vi "testRunCalled.vi"() -> (0 "error out":errorcluster)   [LabVIEW 2019, in "TestSuiteTest.lvlib" / "Run.lvlib"]
uses:
  Run/Run.lvlib
  TestSuite/TestSuite.lvclass
  TestCase/TestCase/TestCase.lvclass
  TestSuiteTestSupport/TestResultMock/TestResultMock.lvclass
  C:/Users/de200256/Code/LVUnit/TestResult/TestResult.lvclass
  Assertion/Assertion.lvlib
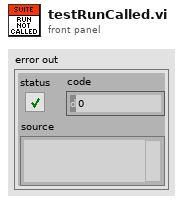
[diagram p1: front panel]
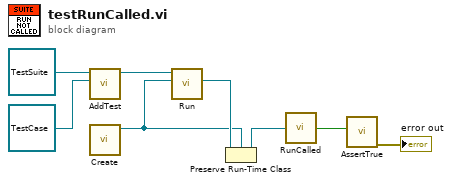
[diagram p0: block diagram]
diagram:
  n1 = call-dynamic "AddTest.vi"("TestCase"=refnum<class "TestCase.lvclass"> refnum, "TestSuite in"=refnum<class "TestSuite.lvclass"> refnum ("TestSuite.lvclass")) -> ("TestSuite out"=w3:refnum<class "TestSuite.lvclass">)  [unwired: 8 in, 1 out]
  n2 = call "Create.vi"() -> ("TestResultMock"=w7:refnum<class "TestResultMock.lvclass">)  [unwired: 10 in, 1 out]
  n3 = call-dynamic "Run.vi"("TestResult"=w7, "TestSuite in"=w3) -> ("TestResult out"=w8:refnum<class "TestResult.lvclass">)  [unwired: 7 in, 2 out]
  n4 = Preserve Run-Time Class(object in=w8, 2:w7) -> (object out=w6:refnum<class "TestResultMock.lvclass">)  [unwired: 1 in, 1 out]
  n5 = call "RunCalled.vi"("TestResultMock In"=w6) -> ("Run Called"=w5:bool)
  n6 = call "AssertTrue.vi"("Condition"=w5) -> ("error out"=→"error out":errorcluster)  [unwired: 10 in]
